vi "Init.vi"(8 "error in (no error)":errorcluster, 11 "uService Template in":refnum<class "Kasli Listener.lvclass">) -> (0 "error out":errorcluster, 3 "uService Template out":refnum<class "Kasli Listener.lvclass">)   [LabVIEW 2020, in "TALOS.lvlib" / "Kasli Listener and Writer.lvlib" / "Kasli Listener.lvclass"]
uses:
  Kasli Listener.lvclass
  C:/LabVIEW Code/TALOS/talos/Ancestor/Ancestor/Ancestor.lvclass
  C:/LabVIEW Code/TALOS/talos/Father of all uServices/Father of all uServices/Father of all uServices.lvclass
  Ancestor/Ancestor/Ancestor.lvclass/Ancestor.ctl
  Father of all uServices/Father of all uServices/Father of all uServices.lvclass/Father of all uServices.ctl
  Support VIs/Substitute Error.vi
  Support VIs/Generate Error.vi
  FGV/Error Memory/Get Error Description.vi
  Support VIs/Get PC name.vi
  Support VIs/Get Class Name.vi
  <vilib>/Utility/error.llb/Clear Errors.vi
  FGV/Error Memory/Error Memory Core.vi
  <vilib>/AdvancedString/Delimited String to 1D String Array.vi
  Support VIs/Circus Root Path.vi
  FGV/Error Memory/Error Crt Lvl checker.vi
  FGV/Error Memory/Error Memory Core.vi/40c8088d-b597-4017-91af-faa98e00292e.vi
  FGV/Error Memory/Error Memory Core.vi/d4a3ab98-063c-4e44-b43d-fbdcfe6c2be2.vi
  Support VIs/Global Memory.vi
  <vilib>/Utility/LVClass/Get LV Class Name.vi
  Support VIs/Is in Packed Library.vi
  Support VIs/TALOS Root path.vi
  Support VIs/Read CSV worksheet.vi
  Support VIs/Global Constants.vi
  <vilib>/Utility/error.llb/General Error Handler.vi
  Support VIs/Error Log.vi
  System uServices/TCP Listener/TCP Listener/TCP Listener.lvclass
  Ancestor/Ancestor/Ancestor.lvclass
  <vilib>/Comparison/Equal/Equal Functor/Equal Functor.lvclass
  Kasli Listener.lvclass/Kasli Listener.ctl
  Father of all uServices/Father of all uServices/Father of all uServices.lvclass
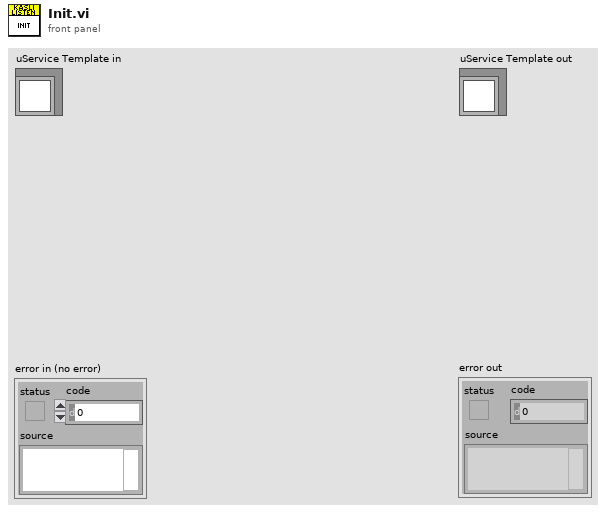
[diagram p1: front panel]
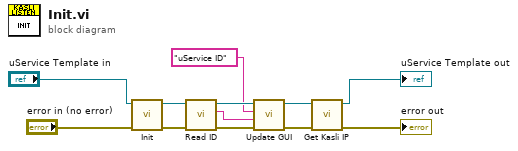
[diagram p0: block diagram]
diagram:
  n1 = call-parent "Init.vi"("error in (no error)"="error in (no error)", "uService Template in"="uService Template in") -> ("error out"=w1:errorcluster, "uService Template out"=w2:refnum<class "Kasli Listener.lvclass">)  [unwired: 8 in]
  n2 = call "Read ID.vi"("error in (no error)"=w1, "Ancestor in"=w2) -> ("error out"=w8:errorcluster, "ID"=w5:string, "Ancestor out"=w7:refnum<class "Kasli Listener.lvclass">)  [unwired: 7 in]
  n3 = call "Update GUI.vi"("error in (no error)"=w8, "Data"=w5, "GUI Item Name"="uService ID", "uService Template in"=w7) -> ("error out"=w3:errorcluster, "uService Template out"=w4:refnum<class "Kasli Listener.lvclass">)  [unwired: 6 in]
  n4 = call "Get Kasli IP.vi"("error in (no error)"=w3, "Kasli Listener in"=w4) -> ("error out"=→"error out":errorcluster, "Kasli Listener out"=→"uService Template out":refnum<class "Kasli Listener.lvclass">)  [unwired: 8 in]
